vi "Call Printer（USB).vi"(2 "写入缓冲区":string, 3 "VISA资源名称":refnum<visa-resource-name>="COM2") -> (0 "error out":errorcluster, 1 "Last P":string)   [LabVIEW 2014]
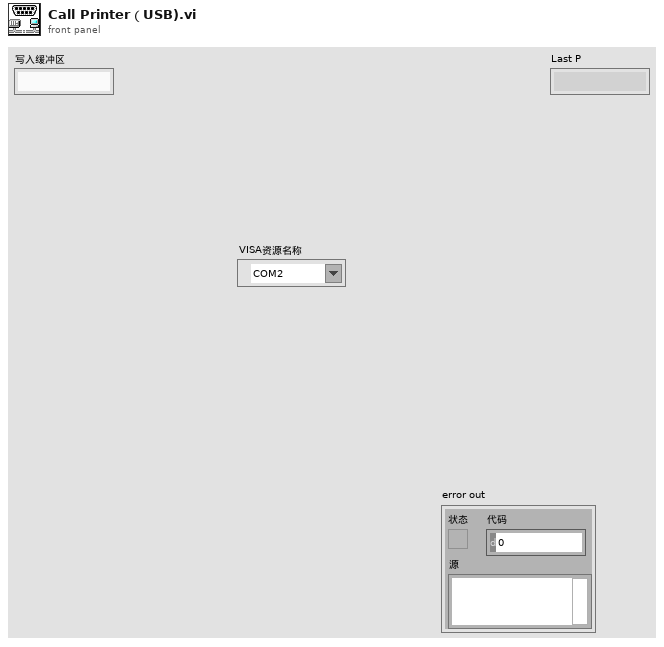
[diagram p1: front panel]
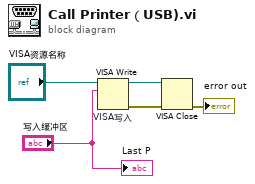
[diagram p0: block diagram]
diagram:
  n1 = VISA Write "VISA写入"(VISA resource name="VISA资源名称", write buffer="写入缓冲区") -> (VISA resource name out=w3:refnum<visa-resource-name>, error out=w2:errorcluster)  [unwired: 1 in, 1 out]
  n2 = VISA Close(VISA resource name=w3, error in (no error)=w2) -> (error out=→"error out":errorcluster)
  "Last P" <- "写入缓冲区"
